vi "Run Bfr Rx - Sized Detect Rollover.vi"(5 "Null Offset":u64, 7 "Buffer Size":u64, 8 "error in (no error)":errorcluster, 11 "Data":u8[](array[numeric])) -> (0 "error out":errorcluster, 1 "Data Size (U64)":u64, 4 "Rollover Occurred?":bool)   [LabVIEW 2016, in "UDP-Custom-Device Engine.lvlib"]
uses:
  UDP-Custom-Device Engine.lvlib
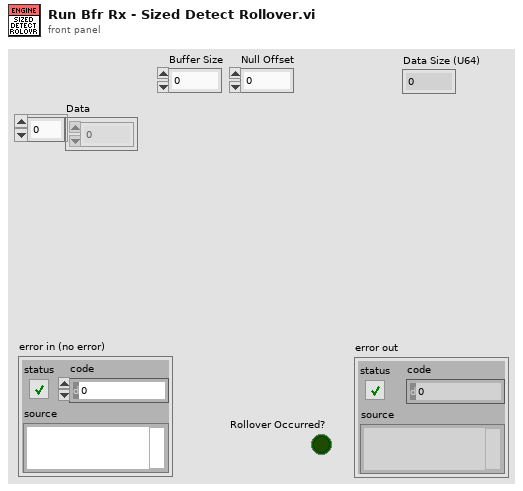
[diagram p1: front panel]
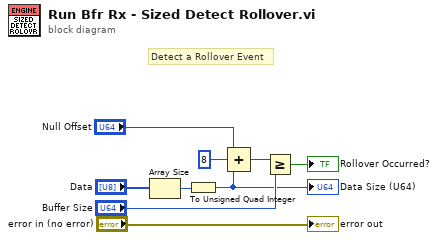
[diagram p0: block diagram]
diagram:
  # "Detect a Rollover Event"
  n1 = Array Size(array="Data") -> (size(s)=w3:i32)
  n2 = To Unsigned Quad Integer(1:w3) -> (0:w1:u64)
  "Data Size (U64)" <- w1
  n3 = Compound Arithmetic op=ADD("Null Offset", u64 8 ("value"), w1) -> (w9:u64)
  n4 = Greater Or Equal?(x=w9, y="Buffer Size") -> (x >= y?=→"Rollover Occurred?":bool)
  "error out" <- "error in (no error)"
